vi "Orifice coefficient For Water.vi"(2 "Water Temperature":dbl[unit]=10.0 min=10.0 max=95.0, 3 "Delta P\n(Presure Made By Orifice)":dbl, 4 "Pipe Diameter (mm)":dbl[unit], 5 "Orifice Diameter":dbl[unit]) -> (0 "Iteration Volumetric Flow \n(Orifice) (Lit/min)":dbl[unit], 1 "Mass Flow (Orifice) (Kg/min)":dbl[unit])   [LabVIEW 2018]
panel:
  out "ReD":dbl
  out "Mass Flow (Orifice) (Kg/h)":dbl[unit](knob)
  out "Mass Flow (Orifice) (Kg/s)":dbl[unit]
  out "Pipe Velocity (m/s)":dbl[unit]
  out "Pipe Area (cm^2)":dbl[unit]
  out "Throat Velocity (m/s)":dbl[unit]
  out "Throat Area (cm^2)":dbl[unit]
  out "Beta":dbl
  out "orifice coefficient":dbl
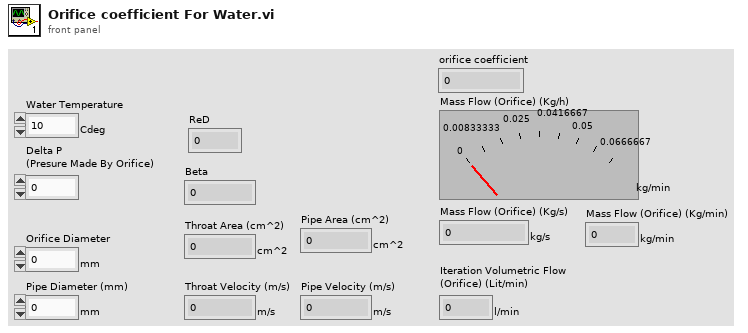
[diagram p1: front panel]
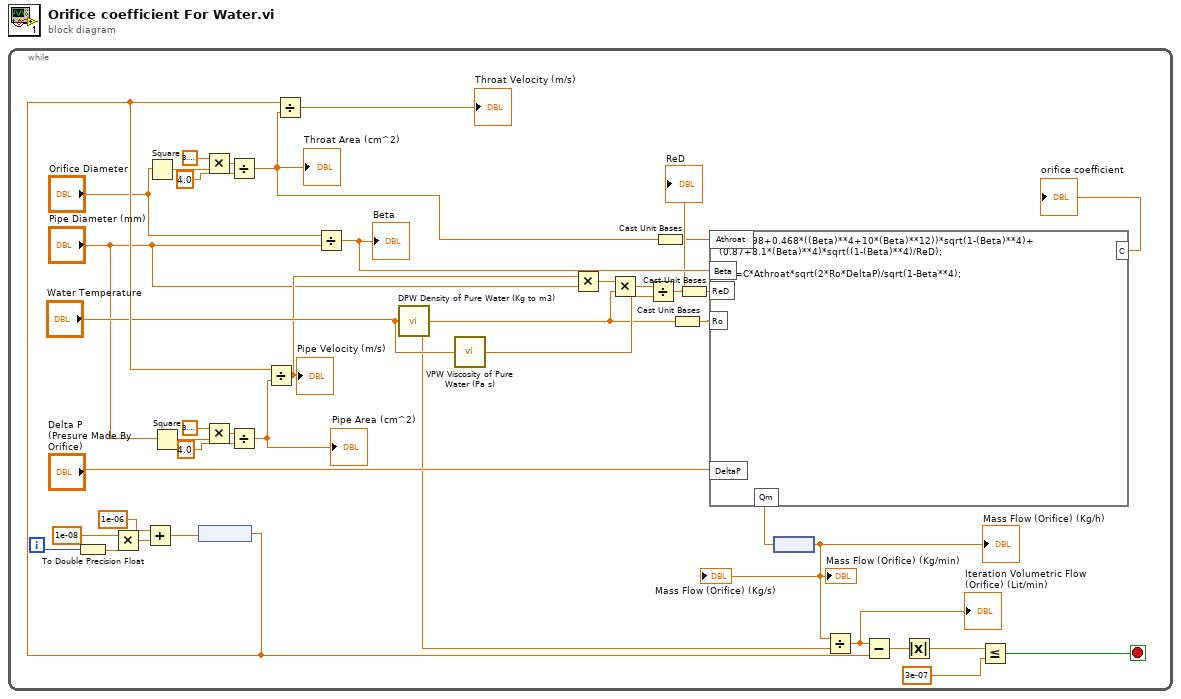
[diagram p0: block diagram]
diagram:
  n1 = while {
    i -> [w23]
    stop <- w16 stop-if-true
    n2 = To Double Precision Float(number=w23) -> (double precision float=w27:dbl)
    n3 = Multiply(x=1e-08, y=w27) -> (x*y=w25:dbl)
    n4 = Add(x=1e-06, y=w25) -> (x+y=w21:dbl)
    n5 = Square(x="Orifice Diameter") -> (x^2=w37:dbl[unit])
    n6 = Square(x="Pipe Diameter (mm)") -> (x^2=w33:dbl[unit])
    n7 = node(w21) -> (w20:dbl[unit])
    n8 = Multiply(x=3.141592653589793, y=w37) -> (x*y=w39:dbl[unit])
    n9 = Multiply(x=3.141592653589793, y=w33) -> (x*y=w35:dbl[unit])
    n10 = Divide(x=w39, y=4.0) -> (x/y=w6:dbl[unit])
    "Throat Area (cm^2)" <- w6
    n11 = Divide(x=w35, y=4.0) -> (x/y=w32:dbl[unit])
    "Pipe Area (cm^2)" <- w32
    n12 = Divide(x=w20, y=w32) -> (x/y=w2:dbl[unit])
    "Pipe Velocity (m/s)" <- w2
    n13 = Divide(x=w20, y=w6) -> (x/y=→"Throat Velocity (m/s)":dbl[unit])
    n14 = Divide(x="Orifice Diameter", y="Pipe Diameter (mm)") -> (x/y=w15:dbl)
    "Beta" <- w15
    n15 = call "DPW Density of Pure Water (Kg to m3).vi"("Pure Water Temprature"="Water Temperature") -> ("DPW"=w3:dbl[unit])
    n16 = call "VPW Viscosity of Pure Water (Pa s).vi"("Pure Water Temprature"="Water Temperature") -> ("Visocity of pure Water (Pa S)"=w8:dbl[unit])
    n17 = Multiply(x=w2, y="Pipe Diameter (mm)") -> (x*y=w14:dbl[unit])
    n18 = Multiply(x=w14, y=w3) -> (x*y=w13:dbl[unit])
    n19 = Divide(x=w13, y=w8) -> (x/y=w10:dbl)
    "ReD" <- w10
    n20 = Cast Unit Bases(0:w6) -> (2:w7:dbl)  [unwired: 1 in]
    n21 = Cast Unit Bases(0:w3) -> (2:w4:dbl)  [unwired: 1 in]
    n22 = Cast Unit Bases(0:w10) -> (2:w9:dbl)  [unwired: 1 in]
    n23 = formula code="C=(0.598+0.468*((Beta)**4+10*(Beta)**12))*sqrt(1-(Beta)**4)+\n(0.87+8.1*(Beta)**4)*sqrt((1-(Beta)**4)/ReD);\n\nQm=C*Athroat*sqrt(2*Ro*DeltaP)/sqrt(1-Beta**4);"("Beta"=w15, "Athroat"=w7, "Ro"=w4, "DeltaP"="Delta P\n(Presure Made By Orifice)", "ReD"=w9) -> ("C"=→"orifice coefficient":dbl, "Qm"=w30:dbl)
    n24 = node(w30) -> (w28:dbl[unit])
    "Mass Flow (Orifice) (Kg/s)" <- w28
    "Mass Flow (Orifice) (Kg/h)" <- w28
    "Mass Flow (Orifice) (Kg/min)" <- w28
    n25 = Divide(x=w28, y=w3) -> (x/y=w22:dbl[unit])
    "Iteration Volumetric Flow \n(Orifice) (Lit/min)" <- w22
    n26 = Subtract(x=w22, y=w20) -> (x-y=w19:dbl[unit])
    n27 = Absolute Value(x=w19) -> (abs(x)=w18:dbl[unit])
    n28 = Less Or Equal?(x=w18, y=dbl[unit] 3e-07) -> (x <= y?=w16:bool)
  }
